vi "Reporting_proc_RMS.vi"(1 "Max RMS Ruedas":dbl[][](array[numeric])) -> (0 "String":string)   [LabVIEW 2015]
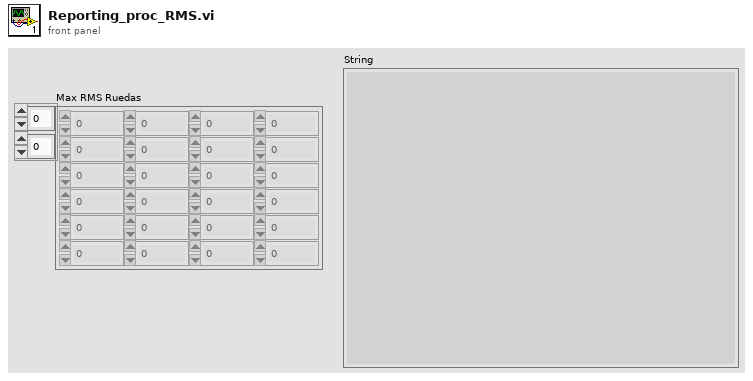
[diagram p1: front panel]
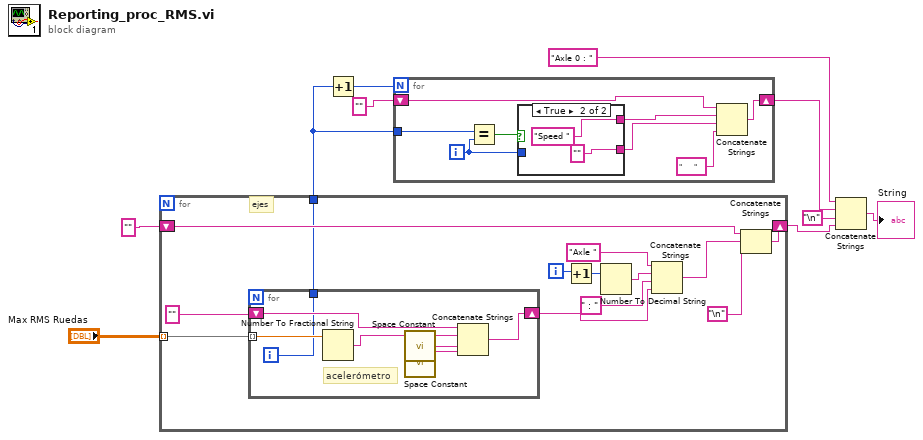
[diagram p0: block diagram]
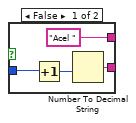
[diagram p2: hidden frame]
diagram:
  n1 = for {
    tunnel: "Max RMS Ruedas" -> [w23] mode=indexing
    shift-right: [w22] -> w4
    shift-left: "" -> [w20]
    tunnel: [w11] -> w1
    i -> [w17]
    # "ejes"
    n2 = for {
      tunnel: w23 -> [w30] mode=indexing
      shift-right: [w26] -> w13
      shift-left: "" -> [w25]
      tunnel: [w24] -> w11
      i -> [w24]
      # "acelerómetro"
      n3 = Number To Fractional String(number=w30) -> (F-format string=w29:string)  [unwired: 3 in]
      n4 = call <vilib>:"Space Constant.vi"() -> ("String"=w28:string)
      n5 = call <vilib>:"Space Constant.vi"() -> ("String"=w27:string)
      n6 = Concatenate Strings(w25, w29, w28, w27) -> (w26:string)
    }
    n7 = Increment(x=w17) -> (x+1=w16:i32)
    n8 = Number To Decimal String(number=w16) -> (decimal integer string=w15:string)  [unwired: 1 in]
    n9 = Concatenate Strings("Axle " ("string"), w15, " : " ("string"), w13) -> (w12:string)
    n10 = Concatenate Strings(w20, w12, "\n") -> (w22:string)
  }
  n11 = Increment(x=w1) -> (x+1=w2:i32)
  n12 = for {
    N: w2 -> [_]
    shift-right: [w35] -> w6
    shift-left: "" -> [w34]
    tunnel: w1 -> [w32]
    i -> [w33]
    n13 = Equal?(x=w32, y=w33) -> (x = y?=w31:bool)
    n14 = case shown="True" w31 {
      tunnel: ["Acel " ("string") "Speed " ("string")] -> w38
      tunnel: [w40 "" ("string")] -> w37
      tunnel: w33 -> [w39 _]
      frame False {
        n15 = Increment(x=w39) -> (x+1=w42:i32)
        n16 = Number To Decimal String(number=w42) -> (decimal integer string=w40:string)  [unwired: 1 in]
      }
      frame True {
      }
    }
    n17 = Concatenate Strings(w34, w38, w37, "      " ("string")) -> (w35:string)
  }
  n18 = Concatenate Strings("Axle 0 : " ("string"), w6, "\n", w4) -> (→"String":string)
